vi "plot_load_sim_output.vi"(6 "Output Files Path":refnum<vi>, 8 "Folder":string, 9 "# Lines Plot":refnum<vi>, 10 "Parameters to Plot":refnum<vi>, 11 "Output File Loaded?":refnum<vi>) -> ()   [LabVIEW 2019]
uses:
  lib/libSimulationControl/libSimulationControl.lvlib
panel:
  # "*******************************************************************\nBiogas Plant Control\n\nAuthor: Paul Zügel\nGCSC-Frankfurt am Main 2020\n\n*******************************************************************"
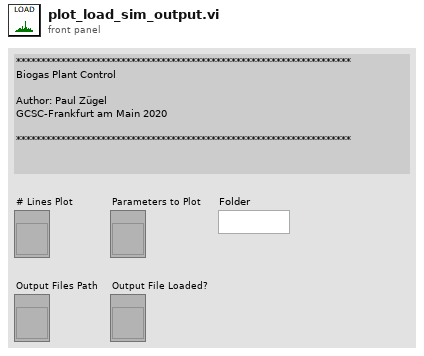
[diagram p1: front panel]
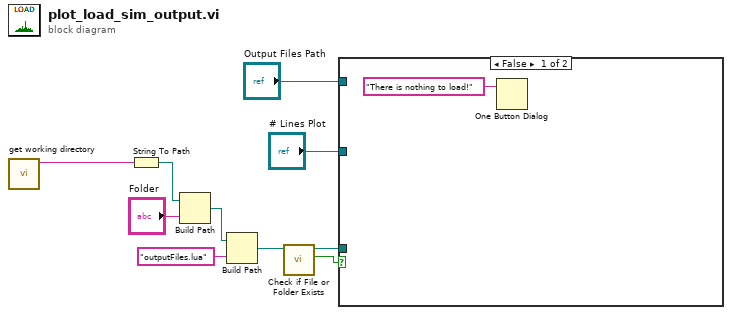
[diagram p0: block diagram]
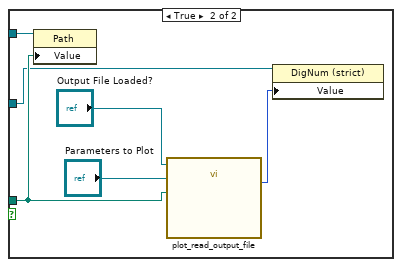
[diagram p2: hidden frame]
diagram:
  n1 = call "get working directory.vi"() -> ("function return"=w3:string)  [unwired: 10 in, 1 out]
  n2 = String To Path(string=w3) -> (path=w1:path)
  n3 = Build Path(base path=w1, name or relative path="Folder") -> (appended path=w2:path)
  n4 = Build Path(base path=w2, name or relative path="outputFiles.lua") -> (appended path=w5:path)
  n5 = call <vilib>:"Check if File or Folder Exists.vi"("path"=w5) -> ("file or folder exists?"=w6:bool, "dup path"=w7:path)  [unwired: 8 in, 1 out]
  n6 = case shown="False" w6 {
    tunnel: w7 -> [_ w14]
    tunnel: "# Lines Plot" -> [_ w13]
    tunnel: "Output Files Path" -> [_ w12]
    frame False {
      n7 = One Button Dialog(message="There is nothing to load!") -> ()  [unwired: 1 in, 1 out]
    }
    frame True {
      n8 = property class="Path"(reference=w12, "Value"=w14) -> ()  [unwired: 1 in, 2 out]
      n9 = call "plot_read_output_file.vi"("TMP Filepath"=w14, "Plot Tree"="Parameters to Plot", "Output File Loaded?"="Output File Loaded?") -> ("# Lines Plot"=w15:i32)  [unwired: 8 in]
      n10 = property class="DigNum (strict)"(reference=w13, "Value"=w15) -> ()  [unwired: 1 in, 2 out]
    }
  }
